vi "GyroSampleSensorLoop.vi"   [LabVIEW 2016]
uses:
  GyroRxLoopData.ctl
  GyroRxLoopStates.ctl
  GyroSBITSample.ctl
  GyroLBITSample.ctl
  GyroSample.ctl
  GyroErrorSample.ctl
  GyroErrorCodes.ctl
  <vilib>/Platform/TimedLoop/XDataNode/timing_clust.ctl
  <vilib>/Platform/TimedLoop/XDataNode/nitl_modes.ctl
  <vilib>/Platform/TimedLoop/XDataNode/wakeup.ctl
  <vilib>/rvi/Emulation/niFpgaSctlEmulationGetInTimedLoop.vi
  <vilib>/rvi/Emulation/niFpgaEmulationReportErrorSimple.vi
  <vilib>/rvi/Emulation/niFpgaGetClockAttributes.vi
  <vilib>/rvi/Emulation/niFpgaCriticalErrorInLSC.vi
  <vilib>/rvi/Emulation/niFpgaEmulationIsFPGAContextNoSignature.vi
  <vilib>/rvi/errors/niFpgaSetErrorForExecOnDevCompSimple.vi
  <vilib>/rvi/eio/common/nirviEmuReportErrorAndStop.vi
  <vilib>/rvi/DataTransferAndStorage/Container/Common/niFpgaContainerGetUniqueNameForEmu.vi
  <vilib>/rvi/FIFO/Fifo_Resource/nirvififoEmulationSetSize.vi
  <vilib>/rvi/FIFO/Fifo_Resource/nirviFifoEmulationQueueMgr.vi
  <instcachedir>/0/nirviFifoEmulationQueueMgr_E5CAEC123FF24DC58D834DCA3CDAA9B5.lvgen/nirviFifoEmulationQueueMgr_E5CAEC123FF24DC58D834DCA3CDAA9B5_009.vi
  <vilib>/Utility/error.llb/Clear Errors.vi
  <vilib>/rvi/FIFO/Fifo_Resource/nirvififoEmulationCreateLock.vi
  <vilib>/rvi/Emulation/niFpgaProcessEmulError.vi
  <vilib>/rvi/FIFO/Fifo_Resource/nirvififoEmulationObtainLock.vi
  <vilib>/rvi/FIFO/Fifo_Resource/nirvififoEmulationReleaseLock.vi
  <vilib>/rvi/occurrence/nirviWaitOnOccurrenceBase.vi
  <vilib>/rvi/errors/nirviReportUnexpectedCaseInternalError.vi
  <vilib>/rvi/errors/nirviReportUnexpectedCaseInternalError (U32).vi
  <vilib>/rvi/FIFO/Fifo_Resource/nirvififoEmulationDetermineInputValidOut.vi
  <vilib>/rvi/Memory/Memory_Emulation/niFpgaMemoryEmulationCacheClearOnFirstRun.vi
  <vilib>/rvi/Memory/Memory_Emulation/nirvimemoryEmulationManagerCache_MakeExclusive.vi
  <vilib>/rvi/Memory/Memory_Emulation/niFpgaMemoryEmulationValidateCache.vi
  <vilib>/rvi/Memory/Memory_Emulation/nirvimemoryEmulationManagerCache_InsertValue.vi
  <vilib>/rvi/Memory/Memory_Emulation/nirvimemoryEmulationManagerCache_ReleaseExclusive.vi
  <vilib>/rvi/Memory/Memory_Emulation/nirvimemoryEmulationManagerCache_GetValue.vi
  <vilib>/rvi/Memory/Memory_Emulation/nirvimemoryEmulationManagerCache_SetValue.vi
  <instcachedir>/0/nirviFifoEmulationQueueMgr_E5CAEC123FF24DC58D834DCA3CDAA9B5.lvgen/nirviFifoEmulationQueueMgr_E5CAEC123FF24DC58D834DCA3CDAA9B5_040.vi
  <instcachedir>/0/nirviFifoEmulationQueueMgr_E5CAEC123FF24DC58D834DCA3CDAA9B5.lvgen/nirviFifoEmulationQueueMgr_E5CAEC123FF24DC58D834DCA3CDAA9B5_041.vi
  <instcachedir>/0/nirviFifoEmulationQueueMgr_E5CAEC123FF24DC58D834DCA3CDAA9B5.lvgen/nirviFifoEmulationQueueMgr_E5CAEC123FF24DC58D834DCA3CDAA9B5_004.vi
  <instcachedir>/0/nirviFifoEmulationQueueMgr_E5CAEC123FF24DC58D834DCA3CDAA9B5.lvgen/nirviFifoEmulationQueueMgr_E5CAEC123FF24DC58D834DCA3CDAA9B5_006.vi
  <instcachedir>/0/nirviFifoEmulationQueueMgr_E5CAEC123FF24DC58D834DCA3CDAA9B5.lvgen/nirviFifoEmulationQueueMgr_E5CAEC123FF24DC58D834DCA3CDAA9B5_042.vi
  <instcachedir>/0/nirviFifoEmulationQueueMgr_E5CAEC123FF24DC58D834DCA3CDAA9B5.lvgen/nirviFifoEmulationQueueMgr_E5CAEC123FF24DC58D834DCA3CDAA9B5_043.vi
  <vilib>/Platform/TimedLoop/XDataNode/XDataNode.xnode
  <vilib>/rvi/DataTransferAndStorage/Container/XNode/niFpgaContainer.xnode
  <vilib>/rvi/FIFO/Fifo_Resource/nirvififoEmulationRead.vi
  <vilib>/rvi/FIFO/Fifo_Resource/nirvififoEmulationWrite.vi
  <vilib>/rvi/DataTransferAndStorage/Register/Emulation/niFpgaRegisterEmulation.vi
  <vilib>/Platform/TimedLoop/XDataNode/XDNodeRunTimeDep.lvlib
types:
  T1 = typedef "GyroRxLoopData.ctl" = cluster{"State":T2, "Timestamp":u64, "Timeout":i32, "CRC":u32, "Checksum":u8, "IsLBIT":bool, "ReservedCount":u8, "SBITSample":T3, "LBITSample":T4, "Sample":T5, "ErrorSample":T6}
  T2 = typedef "GyroRxLoopStates.ctl" = enum16{"ReadHeader3", "IgnoreASCIIResponse", "ReadNormalHeader2", "ReadNormalHeader1", "ReadBITHeader0", "ReadBIT0", "ReadBIT1", "ReadBIT2", "ReadBIT3", "ReadBIT4", "ReadBIT5", "ReadBIT6", "ReadBIT7", "ReadChecksum", "PrepareSBIT", "MoveSBIT", "PrepareLBIT", "MoveLBIT", "ReadSampleHeader0", "ReadSampleX3", "ReadSampleX2", "ReadSampleX1", "ReadSampleX0", "ReadSampleY3", "ReadSampleY2", "ReadSampleY1", "ReadSampleY0", "ReadSampleZ3", "ReadSampleZ2", "ReadSampleZ1", "ReadSampleZ0", "ReadSampleReserved", "ReadSampleStatus", "ReadSampleSequenceNumber", "ReadSampleTemperature1", "ReadSampleTemperature0", "ReadSampleCRC3", "ReadSampleCRC2", "ReadSampleCRC1", "ReadSampleCRC0", "VerifyCRC", "PrepareSample", "MoveSample", "ResponseHeaderError", "ResponseCRCError", "ResponseTimeoutError", "ResponseChecksumError", "PrepareErrorCode", "MoveErrorCode", "ClearCRC", "WaitForCRCCleared"}
  T3 = typedef "GyroSBITSample.ctl" = cluster{"Timestamp":u64, "TxBytes":u64, "RxBytes":u64, "TxFrames":u64, "RxFrames":u64, "BIT0":u8, "BIT1":u8, "BIT2":u8, "BIT3":u8, "BIT4":u8, "BIT5":u8}
  T4 = typedef "GyroLBITSample.ctl" = cluster{"Timestamp":u64, "TxBytes":u64, "RxBytes":u64, "TxFrames":u64, "RxFrames":u64, "BIT0":u8, "BIT1":u8, "BIT2":u8, "BIT3":u8, "BIT4":u8, "BIT5":u8, "BIT6":u8, "BIT7":u8}
  T5 = typedef "GyroSample.ctl" = cluster{"Timestamp":u64, "TxBytes":u64, "RxBytes":u64, "TxFrames":u64, "RxFrames":u64, "GyroX":u32, "GyroY":u32, "GyroZ":u32, "Status":u8, "SequenceNumber":u8, "Temperature":i16}
  T6 = typedef "GyroErrorSample.ctl" = cluster{"Timestamp":u64, "TxBytes":u64, "RxBytes":u64, "TxFrames":u64, "RxFrames":u64, "ErrorCode":T7}
  T7 = typedef "GyroErrorCodes.ctl" = enum8{"None", "ResponseHeaderError", "ResponseCRCError", "ResponseTimeoutError", "ResponseChecksumError"}
  T8 = typedef "XDNodeRunTimeDep.lvlib/timing_clust.ctl" = cluster{"Expected End [f-1]":u64, "Actual End [f-1]":u64, "Finished Late? [f-1]":bool, "Expected End [i-1]":u64, "Actual End [i-1]":u64, "Finished Late? [i-1]":bool, "Expected Start [i]":u64, "Actual Start [i]":u64, "Expected Start [f]":u64, "Actual Start [f]":u64, "Source Name":string, "Structure Name":string, "Period":i64, "Deadline":i64, "Offset":i64, "Start":i64, "Priority":i32, "Timeout":i32, "Mode":T9, "Wakeup Reason":T10, "Error":errorcluster, "Source Type":string, "Secondary Source Type":string, "Global End Time":u64, "Global Start Time":u64, "Frame Duration":u64, "Iteration Duration":u64, "Assigned CPU":i32, "I/O Scan Engine Mode":u32}
  T9 = typedef "XDNodeRunTimeDep.lvlib/nitl_modes.ctl" = enum32{"No Change", "Process missed periods, maintain original phase", "Discard missed periods, maintain original phase", "Process missed periods, ignore original phase", "Discard missed periods, ignore original phase"}
  T10 = typedef "XDNodeRunTimeDep.lvlib/wakeup.ctl" = enum32{"Normal", "Aborted", "Asynchronous wakeup", "Timing source error", "Timed loop error", "Timeout"}
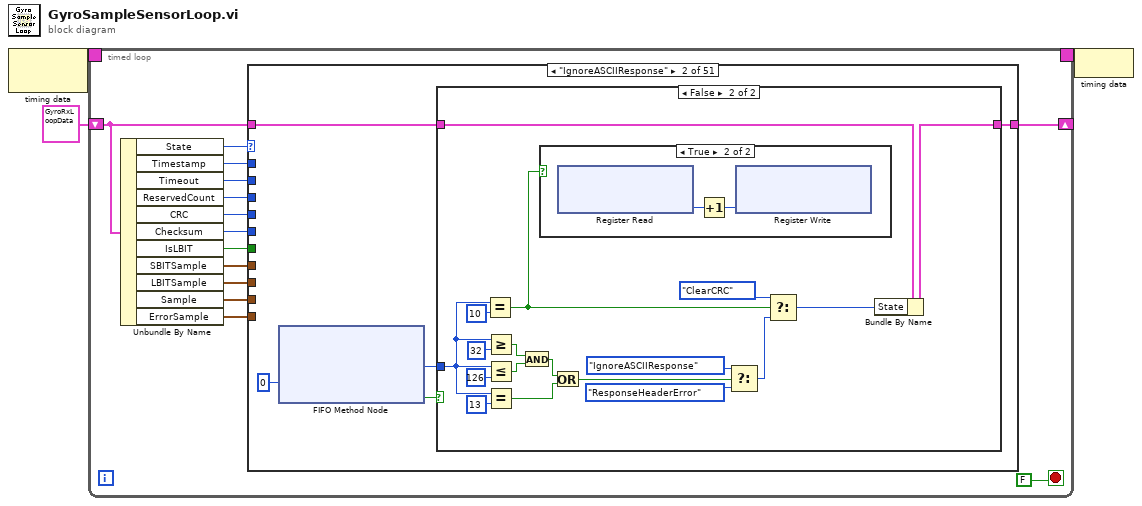
[diagram p0: block diagram]
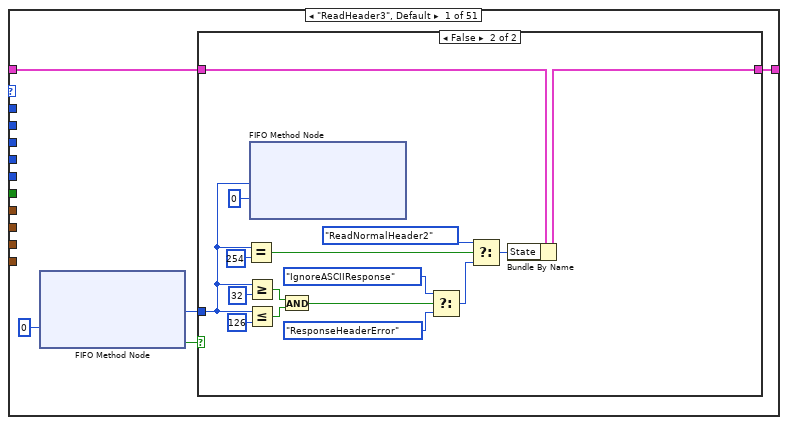
[diagram p2: hidden frame]
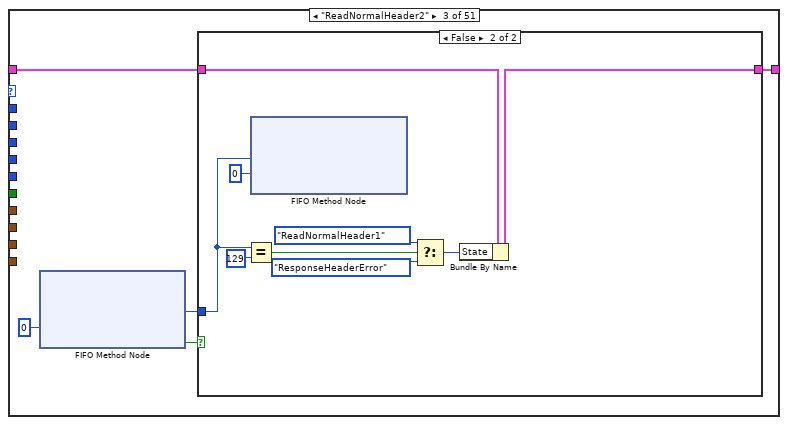
[diagram p6: hidden frame]
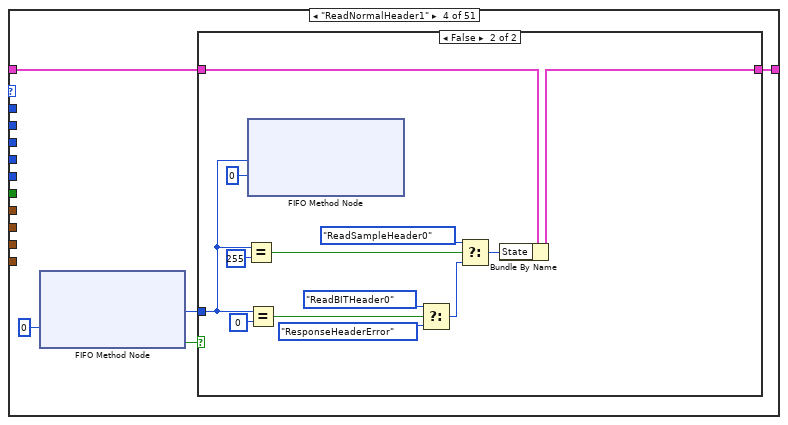
[diagram p8: hidden frame]
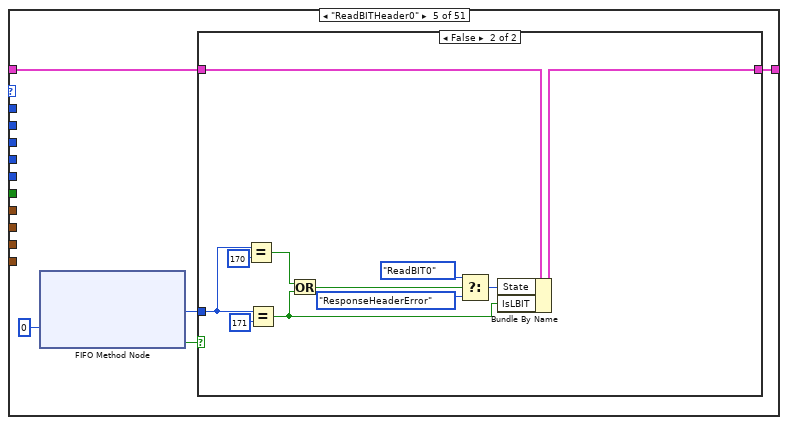
[diagram p10: hidden frame]
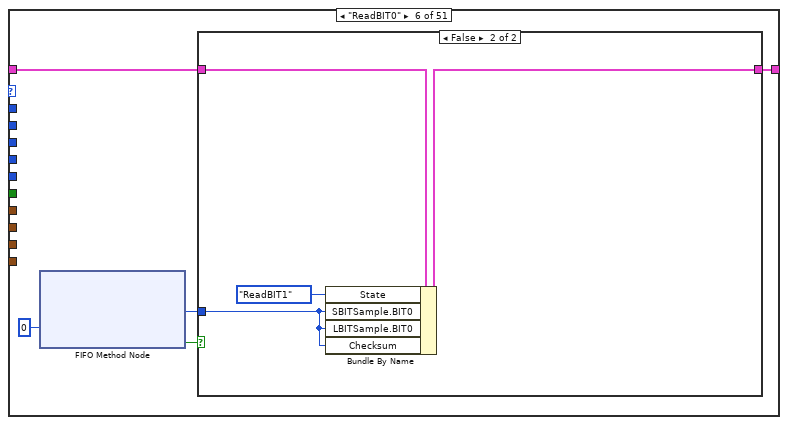
[diagram p12: hidden frame]
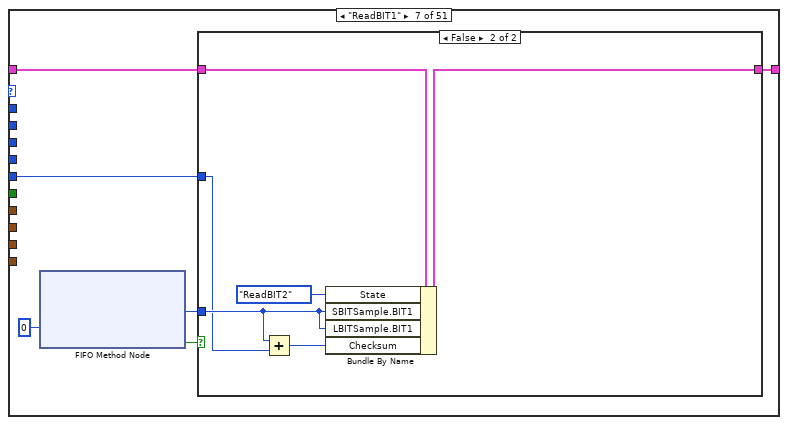
[diagram p14: hidden frame]
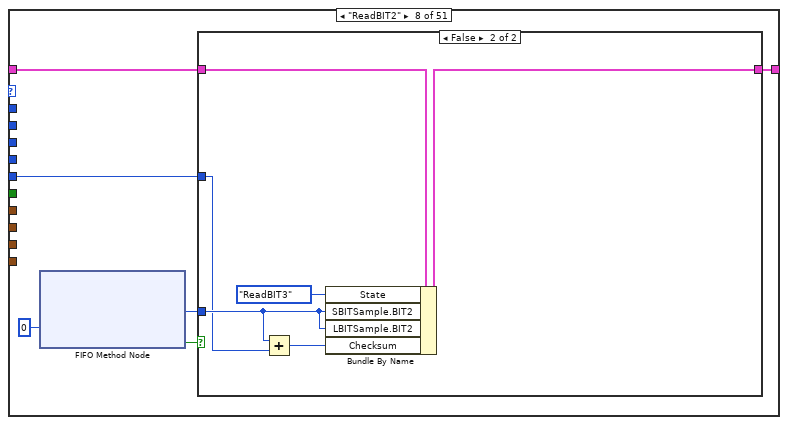
[diagram p16: hidden frame]
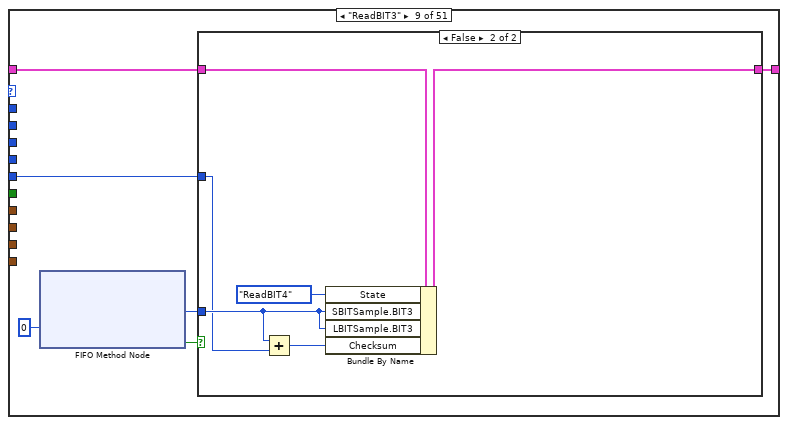
[diagram p18: hidden frame]
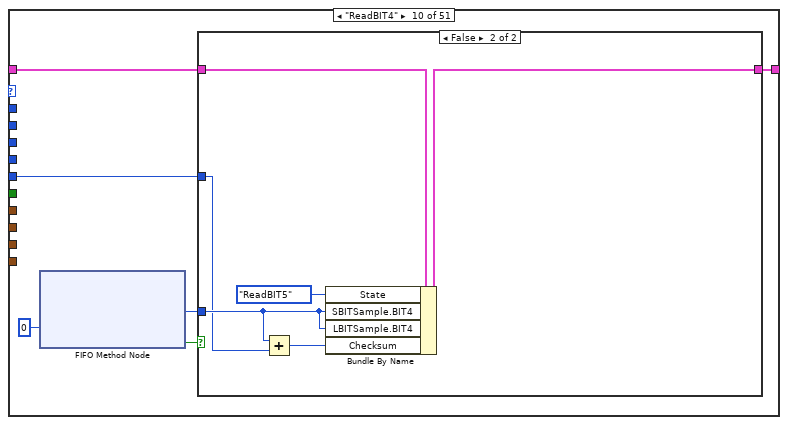
[diagram p20: hidden frame]
diagram:
  n1 = node-c288() -> (w3:T8)  [unwired: 1 in]
  n2 = timed-loop {
    timing: w3 -> [_]
    timing-out: [_] -> w2
    shift-right: [w17] -> _
    shift-left: T1 {"State"=enum."ReadHeader3", "Timestamp"=0, "Timeout"=0, "CRC"=0, "Checksum"=0, "IsLBIT"=FALSE, "ReservedCount"=0, "SBITSample"={"Timestamp"=0, "TxBytes"=0, "RxBytes"=0, "TxFrames"=0, "RxFrames"=0, "BIT0"=0, "BIT1"=0, "BIT2"=0, "BIT3"=0, "BIT4"=0, "BIT5"=0}, "LBITSample"={"Timestamp"=0, "TxBytes"=0, "RxBytes"=0, "TxFrames"=0, "RxFrames"=0, "BIT0"=0, "BIT1"=0, "BIT2"=0, "BIT3"=0, "BIT4"=0, "BIT5"=0, "BIT6"=0, "BIT7"=0}, "Sample"={"Timestamp"=0, "TxBytes"=0, "RxBytes"=0, "TxFrames"=0, "RxFrames"=0, "GyroX"=0, "GyroY"=0, "GyroZ"=0, "Status"=0, "SequenceNumber"=0, "Temperature"=0}, "ErrorSample"={"Timestamp"=0, "TxBytes"=0, "RxBytes"=0, "TxFrames"=0, "RxFrames"=0, "ErrorCode"=enum."None"}} ("GyroRxLoopData") -> [w16]
    stop <- FALSE stop-if-true
    n3 = Unbundle By Name(w16) -> ("State"=w15:T2, "Timestamp"=w14:u64, "Timeout"=w13:i32, "ReservedCount"=w9:u8, "CRC"=w12:u32, "Checksum"=w11:u8, "IsLBIT"=w10:bool, "SBITSample"=w8:T3, "LBITSample"=w7:T4, "Sample"=w6:T5, "ErrorSample"=w5:T6)
    n4 = case shown="\"IgnoreASCIIResponse\"" w15 {
      tunnel: [w18 w40 w66 w81 w100 w117 w128 w141 w154 w167 w181 w197 w210 w224 w249 w254 w262 w267 w269 w284 w298 w314 w330 w344 w358 w374 w390 w404 w418 w434 w450 w466 w483 w494 w505 w519 w533 w549 w565 w581 w595 w617 w622 w626 w630 w634 w638 w646 w651 w656 w663] -> w17
      tunnel: w16 -> [w19 w41 w67 w82 w101 w118 w129 w142 w155 w168 w182 w198 w211 w225 w250 w255 w263 w268 w270 w285 w299 w315 w331 w345 w359 w375 w391 w405 w419 w435 w451 w467 w484 w495 w506 w520 w534 w550 w566 w582 w596 w618 w623 w627 w631 w635 w639 w647 w652 w657 w664]
      tunnel: w14 -> [_ _ _ _ _ _ _ _ _ _ _ _ _ _ w247 _ w260 _ _ _ _ _ _ _ _ _ _ _ _ _ _ _ _ _ _ _ _ _ _ _ _ w615 _ _ _ _ _ w644 _ _ _]
      tunnel: w13 -> [_ _ _ _ _ _ _ _ _ _ _ _ _ _ _ _ _ _ _ _ _ _ _ _ _ _ _ _ _ _ _ _ _ _ _ _ _ _ _ _ _ _ _ _ _ _ _ _ _ _ _]
      tunnel: w12 -> [_ _ _ _ _ _ _ _ _ _ _ _ _ _ _ _ _ _ _ _ _ _ _ _ _ _ _ _ _ _ _ _ _ _ _ _ _ w548 w564 w580 w594 _ _ _ _ _ _ _ _ _ _]
      tunnel: w11 -> [_ _ _ _ _ _ w127 w140 w153 w166 w180 w196 w209 w223 _ _ _ _ _ _ _ _ _ _ _ _ _ _ _ _ _ _ _ _ _ _ _ _ _ _ _ _ _ _ _ _ _ _ _ _ _]
      tunnel: w10 -> [_ _ _ _ _ _ _ _ _ _ w179 _ _ w222 _ _ _ _ _ _ _ _ _ _ _ _ _ _ _ _ _ _ _ _ _ _ _ _ _ _ _ _ _ _ _ _ _ _ _ _ _]
      tunnel: w9 -> [_ _ _ _ _ _ _ _ _ _ _ _ _ _ _ _ _ _ _ _ _ _ _ _ _ _ _ _ _ _ _ w465 _ _ _ _ _ _ _ _ _ _ _ _ _ _ _ _ _ _ _]
      tunnel: w8 -> [_ _ _ _ _ _ _ _ _ _ _ _ _ _ _ w251 _ _ _ _ _ _ _ _ _ _ _ _ _ _ _ _ _ _ _ _ _ _ _ _ _ _ _ _ _ _ _ _ _ _ _]
      tunnel: w7 -> [_ _ _ _ _ _ _ _ _ _ _ _ _ _ _ _ _ w264 _ _ _ _ _ _ _ _ _ _ _ _ _ _ _ _ _ _ _ _ _ _ _ _ _ _ _ _ _ _ _ _ _]
      tunnel: w6 -> [_ _ _ _ _ _ _ _ _ _ _ _ _ _ _ _ _ _ _ _ _ _ _ _ _ _ _ _ _ _ _ _ _ _ _ _ _ _ _ _ _ _ w620 _ _ _ _ _ _ _ _]
      tunnel: w5 -> [_ _ _ _ _ _ _ _ _ _ _ _ _ _ _ _ _ _ _ _ _ _ _ _ _ _ _ _ _ _ _ _ _ _ _ _ _ _ _ _ _ _ _ _ _ _ _ _ w649 _ _]
      frame "ReadHeader3", Default {
        n5 = xnode ("FIFO Method Node")("Timeout"=0) -> ("Element"=w21:u8, "Timed Out?"=w20:bool)  [unwired: 1 in, 1 out]
        n6 = case shown="False" w20 {
          tunnel: w21 -> [_ w25]
          tunnel: w19 -> [w23 w28]
          tunnel: [w23 w27] -> w18
          frame True {
          }
          frame False {
            n7 = Equal?(x=w25, y=u8 254) -> (x = y?=w29:bool)
            n8 = Greater Or Equal?(x=w25, y=u8 32) -> (x >= y?=w36:bool)
            n9 = Less Or Equal?(x=w25, y=u8 126) -> (x <= y?=w35:bool)
            n10 = xnode ("FIFO Method Node")("Element"=w25, "Timeout"=0) -> ()  [unwired: 1 in, 2 out]
            n11 = And(x=w36, y=w35) -> (x .and. y?=w34:bool)
            n12 = Select(t=GyroRxLoopStates."IgnoreASCIIResponse", s=w34, f=GyroRxLoopStates."ResponseHeaderError" ("GyroRxLoopStates")) -> (s? t:f=w33:T2)
            n13 = Select(t=GyroRxLoopStates."ReadNormalHeader2", s=w29, f=w33) -> (s? t:f=w26:T2)
            n14 = Bundle By Name(cluster=w28, "State"=w26) -> (w27:T1)
          }
        }
      }
      frame "IgnoreASCIIResponse" {
        n15 = xnode ("FIFO Method Node")("Timeout"=0) -> ("Element"=w43:u8, "Timed Out?"=w42:bool)  [unwired: 1 in, 1 out]
        n16 = case shown="False" w42 {
          tunnel: w43 -> [_ w55]
          tunnel: w41 -> [w45 w59]
          tunnel: [w45 w58] -> w40
          frame True {
          }
          frame False {
            n17 = Equal?(x=w55, y=u8 10) -> (x = y?=w46:bool)
            n18 = Greater Or Equal?(x=w55, y=u8 32) -> (x >= y?=w54:bool)
            n19 = Less Or Equal?(x=w55, y=u8 126) -> (x <= y?=w53:bool)
            n20 = Equal?(x=w55, y=u8 13) -> (x = y?=w51:bool)
            n21 = And(x=w54, y=w53) -> (x .and. y?=w52:bool)
            n22 = case shown="True" w46 {
              frame False {
              }
              frame True {
                n23 = xnode ("Register Read")() -> ("Data"=w65:u64)  [unwired: 1 in, 1 out]
                n24 = Increment(x=w65) -> (x+1=w64:u64)
                n25 = xnode ("Register Write")("Data"=w64) -> ()  [unwired: 1 in, 1 out]
              }
            }
            n26 = Or(x=w52, y=w51) -> (x .or. y?=w50:bool)
            n27 = Select(t=GyroRxLoopStates."IgnoreASCIIResponse", s=w50, f=GyroRxLoopStates."ResponseHeaderError" ("t")) -> (s? t:f=w47:T2)
            n28 = Select(t=GyroRxLoopStates."ClearCRC", s=w46, f=w47) -> (s? t:f=w57:T2)
            n29 = Bundle By Name(cluster=w59, "State"=w57) -> (w58:T1)
          }
        }
      }
      frame "ReadNormalHeader2" {
        n30 = xnode ("FIFO Method Node")("Timeout"=0) -> ("Element"=w69:u8, "Timed Out?"=w68:bool)  [unwired: 1 in, 1 out]
        n31 = case shown="False" w68 {
          tunnel: w69 -> [_ w72]
          tunnel: w67 -> [w71 w77]
          tunnel: [w71 w76] -> w66
          frame True {
          }
          frame False {
            n32 = Equal?(x=w72, y=u8 129) -> (x = y?=w78:bool)
            n33 = xnode ("FIFO Method Node")("Element"=w72, "Timeout"=0) -> ()  [unwired: 1 in, 2 out]
            n34 = Select(t=GyroRxLoopStates."ReadNormalHeader1", s=w78, f=GyroRxLoopStates."ResponseHeaderError") -> (s? t:f=w75:T2)
            n35 = Bundle By Name(cluster=w77, "State"=w75) -> (w76:T1)
          }
        }
      }
      frame "ReadNormalHeader1" {
        n36 = xnode ("FIFO Method Node")("Timeout"=0) -> ("Element"=w84:u8, "Timed Out?"=w83:bool)  [unwired: 1 in, 1 out]
        n37 = case shown="False" w83 {
          tunnel: w84 -> [_ w87]
          tunnel: w82 -> [w86 w96]
          tunnel: [w86 w95] -> w81
          frame True {
          }
          frame False {
            n38 = Equal?(x=w87, y=u8 255) -> (x = y?=w97:bool)
            n39 = xnode ("FIFO Method Node")("Element"=w87, "Timeout"=0) -> ()  [unwired: 1 in, 2 out]
            n40 = Equal?(x=w87, y=u8 0) -> (x = y?=w92:bool)
            n41 = Select(t=GyroRxLoopStates."ReadBITHeader0" ("f"), s=w92, f=GyroRxLoopStates."ResponseHeaderError") -> (s? t:f=w89:T2)
            n42 = Select(t=GyroRxLoopStates."ReadSampleHeader0", s=w97, f=w89) -> (s? t:f=w94:T2)
            n43 = Bundle By Name(cluster=w96, "State"=w94) -> (w95:T1)
          }
        }
      }
      frame "ReadBITHeader0" {
        n44 = xnode ("FIFO Method Node")("Timeout"=0) -> ("Element"=w103:u8, "Timed Out?"=w102:bool)  [unwired: 1 in, 1 out]
        n45 = case shown="False" w102 {
          tunnel: w103 -> [_ w110]
          tunnel: w101 -> [w105 w114]
          tunnel: [w105 w113] -> w100
          frame True {
          }
          frame False {
            n46 = Equal?(x=w110, y=u8 170) -> (x = y?=w109:bool)
            n47 = Equal?(x=w110, y=u8 171) -> (x = y?=w107:bool)
            n48 = Or(x=w109, y=w107) -> (x .or. y?=w108:bool)
            n49 = Select(t=GyroRxLoopStates."ReadBIT0", s=w108, f=GyroRxLoopStates."ResponseHeaderError") -> (s? t:f=w112:T2)
            n50 = Bundle By Name(cluster=w114, "State"=w112, "IsLBIT"=w107) -> (w113:T1)
          }
        }
      }
      frame "ReadBIT0" {
        n51 = xnode ("FIFO Method Node")("Timeout"=0) -> ("Element"=w120:u8, "Timed Out?"=w119:bool)  [unwired: 1 in, 1 out]
        n52 = case shown="False" w119 {
          tunnel: w120 -> [_ w123]
          tunnel: w118 -> [w122 w126]
          tunnel: [w122 w125] -> w117
          frame True {
          }
          frame False {
            n53 = Bundle By Name(cluster=w126, "State"=GyroRxLoopStates."ReadBIT1" ("t"), "SBITSample.BIT0"=w123, "LBITSample.BIT0"=w123, "Checksum"=w123) -> (w125:T1)
          }
        }
      }
      frame "ReadBIT1" {
        n54 = xnode ("FIFO Method Node")("Timeout"=0) -> ("Element"=w131:u8, "Timed Out?"=w130:bool)  [unwired: 1 in, 1 out]
        n55 = case shown="False" w130 {
          tunnel: w131 -> [_ w136]
          tunnel: w129 -> [w133 w139]
          tunnel: [w133 w138] -> w128
          tunnel: w127 -> [_ w135]
          frame True {
          }
          frame False {
            n56 = Add(x=w136, y=w135) -> (x+y=w134:u8)
            n57 = Bundle By Name(cluster=w139, "State"=GyroRxLoopStates."ReadBIT2" ("t"), "SBITSample.BIT1"=w136, "LBITSample.BIT1"=w136, "Checksum"=w134) -> (w138:T1)
          }
        }
      }
      frame "ReadBIT2" {
        n58 = xnode ("FIFO Method Node")("Timeout"=0) -> ("Element"=w144:u8, "Timed Out?"=w143:bool)  [unwired: 1 in, 1 out]
        n59 = case shown="False" w143 {
          tunnel: w144 -> [_ w149]
          tunnel: w142 -> [w146 w152]
          tunnel: [w146 w151] -> w141
          tunnel: w140 -> [_ w148]
          frame True {
          }
          frame False {
            n60 = Add(x=w149, y=w148) -> (x+y=w147:u8)
            n61 = Bundle By Name(cluster=w152, "State"=GyroRxLoopStates."ReadBIT3" ("t"), "SBITSample.BIT2"=w149, "LBITSample.BIT2"=w149, "Checksum"=w147) -> (w151:T1)
          }
        }
      }
      frame "ReadBIT3" {
        n62 = xnode ("FIFO Method Node")("Timeout"=0) -> ("Element"=w157:u8, "Timed Out?"=w156:bool)  [unwired: 1 in, 1 out]
        n63 = case shown="False" w156 {
          tunnel: w157 -> [_ w162]
          tunnel: w155 -> [w159 w165]
          tunnel: [w159 w164] -> w154
          tunnel: w153 -> [_ w161]
          frame True {
          }
          frame False {
            n64 = Add(x=w162, y=w161) -> (x+y=w160:u8)
            n65 = Bundle By Name(cluster=w165, "State"=GyroRxLoopStates."ReadBIT4" ("t"), "SBITSample.BIT3"=w162, "LBITSample.BIT3"=w162, "Checksum"=w160) -> (w164:T1)
          }
        }
      }
      frame "ReadBIT4" {
        n66 = xnode ("FIFO Method Node")("Timeout"=0) -> ("Element"=w170:u8, "Timed Out?"=w169:bool)  [unwired: 1 in, 1 out]
        n67 = case shown="False" w169 {
          tunnel: w170 -> [_ w175]
          tunnel: w168 -> [w172 w178]
          tunnel: [w172 w177] -> w167
          tunnel: w166 -> [_ w174]
          frame True {
          }
          frame False {
            n68 = Add(x=w175, y=w174) -> (x+y=w173:u8)
            n69 = Bundle By Name(cluster=w178, "State"=GyroRxLoopStates."ReadBIT5" ("t"), "SBITSample.BIT4"=w175, "LBITSample.BIT4"=w175, "Checksum"=w173) -> (w177:T1)
          }
        }
      }
      frame "ReadBIT5" {
        n70 = xnode ("FIFO Method Node")("Timeout"=0) -> ("Element"=w184:u8, "Timed Out?"=w183:bool)  [unwired: 1 in, 1 out]
        n71 = case shown="False" w183 {
          tunnel: w184 -> [_ w193]
          tunnel: w182 -> [w186 w195]
          tunnel: [w186 w194] -> w181
          tunnel: w180 -> [_ w192]
          tunnel: w179 -> [_ w190]
          frame True {
          }
          frame False {
            n72 = Add(x=w193, y=w192) -> (x+y=w191:u8)
            n73 = Select(t=GyroRxLoopStates."ReadBIT6", s=w190, f=GyroRxLoopStates."ReadChecksum") -> (s? t:f=w187:T2)
            n74 = Bundle By Name(cluster=w195, "State"=w187, "SBITSample.BIT5"=w193, "LBITSample.BIT5"=w193, "Checksum"=w191) -> (w194:T1)
          }
        }
      }
      frame "ReadBIT6" {
        n75 = xnode ("FIFO Method Node")("Timeout"=0) -> ("Element"=w200:u8, "Timed Out?"=w199:bool)  [unwired: 1 in, 1 out]
        n76 = case shown="False" w199 {
          tunnel: w200 -> [_ w206]
          tunnel: w198 -> [w202 w208]
          tunnel: [w202 w207] -> w197
          tunnel: w196 -> [_ w205]
          frame True {
          }
          frame False {
            n77 = Add(x=w206, y=w205) -> (x+y=w204:u8)
            n78 = Bundle By Name(cluster=w208, "State"=GyroRxLoopStates."ReadBIT7" ("t"), "LBITSample.BIT6"=w206, "Checksum"=w204) -> (w207:T1)
          }
        }
      }
      frame "ReadBIT7" {
        n79 = xnode ("FIFO Method Node")("Timeout"=0) -> ("Element"=w213:u8, "Timed Out?"=w212:bool)  [unwired: 1 in, 1 out]
        n80 = case shown="False" w212 {
          tunnel: w213 -> [_ w219]
          tunnel: w211 -> [w215 w221]
          tunnel: [w215 w220] -> w210
          tunnel: w209 -> [_ w218]
          frame True {
          }
          frame False {
            n81 = Add(x=w219, y=w218) -> (x+y=w217:u8)
            n82 = Bundle By Name(cluster=w221, "State"=GyroRxLoopStates."ReadChecksum" ("t"), "LBITSample.BIT7"=w219, "Checksum"=w217) -> (w220:T1)
          }
        }
      }
      frame "ReadChecksum" {
        n83 = xnode ("FIFO Method Node")("Timeout"=0) -> ("Element"=w227:u8, "Timed Out?"=w226:bool)  [unwired: 1 in, 1 out]
        n84 = case shown="False" w226 {
          tunnel: w227 -> [_ w238]
          tunnel: w225 -> [w229 w240]
          tunnel: [w229 w239] -> w224
          tunnel: w223 -> [_ w237]
          tunnel: w222 -> [_ w236]
          frame True {
          }
          frame False {
            n85 = Not Equal?(x=w237, y=w238) -> (x != y?=w230:bool)
            n86 = Select(t=GyroRxLoopStates."PrepareLBIT", s=w236, f=GyroRxLoopStates."PrepareSBIT" ("t")) -> (s? t:f=w232:T2)
            n87 = case shown="False" w230 {
              frame True {
              }
              frame False {
                n88 = xnode ("Register Read")() -> ("Data"=w242:u64)  [unwired: 1 in, 1 out]
                n89 = Increment(x=w242) -> (x+1=w241:u64)
                n90 = xnode ("Register Write")("Data"=w241) -> ()  [unwired: 1 in, 1 out]
              }
            }
            n91 = Select(t=GyroRxLoopStates."ResponseChecksumError", s=w230, f=w232) -> (s? t:f=w231:T2)
            n92 = Bundle By Name(cluster=w240, "State"=w231) -> (w239:T1)
          }
        }
      }
      frame "PrepareSBIT" {
        n93 = xnode ("Register Read")() -> ("Data"=w246:u64)  [unwired: 1 in, 1 out]
        n94 = xnode ("Register Read")() -> ("Data"=w245:u64)  [unwired: 1 in, 1 out]
        n95 = xnode ("Register Read")() -> ("Data"=w244:u64)  [unwired: 1 in, 1 out]
        n96 = xnode ("Register Read")() -> ("Data"=w243:u64)  [unwired: 1 in, 1 out]
        n97 = Bundle By Name(cluster=w250, "State"=GyroRxLoopStates."MoveSBIT", "SBITSample.Timestamp"=w247, "SBITSample.TxBytes"=w246, "SBITSample.RxBytes"=w245, "SBITSample.TxFrames"=w244, "SBITSample.RxFrames"=w243) -> (w249:T1)
      }
      frame "MoveSBIT" {
        n98 = xnode ("FIFO Method Node")("Element"=w251, "Timeout"=0) -> ()  [unwired: 1 in, 2 out]
        n99 = Bundle By Name(cluster=w255, "State"=GyroRxLoopStates."ClearCRC") -> (w254:T1)
      }
      frame "PrepareLBIT" {
        n100 = xnode ("Register Read")() -> ("Data"=w259:u64)  [unwired: 1 in, 1 out]
        n101 = xnode ("Register Read")() -> ("Data"=w258:u64)  [unwired: 1 in, 1 out]
        n102 = xnode ("Register Read")() -> ("Data"=w257:u64)  [unwired: 1 in, 1 out]
        n103 = xnode ("Register Read")() -> ("Data"=w256:u64)  [unwired: 1 in, 1 out]
        n104 = Bundle By Name(cluster=w263, "State"=GyroRxLoopStates."MoveLBIT", "LBITSample.Timestamp"=w260, "LBITSample.TxBytes"=w259, "LBITSample.RxBytes"=w258, "LBITSample.TxFrames"=w257, "LBITSample.RxFrames"=w256) -> (w262:T1)
      }
      frame "MoveLBIT" {
        n105 = xnode ("FIFO Method Node")("Element"=w264, "Timeout"=0) -> ()  [unwired: 1 in, 2 out]
        n106 = Bundle By Name(cluster=w268, "State"=GyroRxLoopStates."ClearCRC") -> (w267:T1)
      }
      frame "ReadSampleHeader0" {
        n107 = xnode ("FIFO Method Node")("Timeout"=0) -> ("Element"=w272:u8, "Timed Out?"=w271:bool)  [unwired: 1 in, 1 out]
        n108 = case shown="False" w271 {
          tunnel: w272 -> [_ w275]
          tunnel: w270 -> [w274 w281]
          tunnel: [w274 w280] -> w269
          frame True {
          }
          frame False {
            n109 = xnode ("FIFO Method Node")("Element"=w275, "Timeout"=0) -> ()  [unwired: 1 in, 2 out]
            n110 = Equal?(x=w275, y=u8 85) -> (x = y?=w277:bool)
            n111 = Select(t=GyroRxLoopStates."ReadSampleX3", s=w277, f=GyroRxLoopStates."ResponseHeaderError") -> (s? t:f=w279:T2)
            n112 = Bundle By Name(cluster=w281, "State"=w279) -> (w280:T1)
          }
        }
      }
      frame "ReadSampleX3" {
        n113 = xnode ("FIFO Method Node")("Timeout"=0) -> ("Element"=w287:u8, "Timed Out?"=w286:bool)  [unwired: 1 in, 1 out]
        n114 = case shown="False" w286 {
          tunnel: w287 -> [_ w294]
          tunnel: w285 -> [w289 w291]
          tunnel: [w289 w297] -> w284
          frame True {
          }
          frame False {
            n115 = To Unsigned Long Integer(number=w294) -> (unsigned 32bit integer=w293:u32)
            n116 = xnode ("FIFO Method Node")("Element"=w294, "Timeout"=0) -> ()  [unwired: 1 in, 2 out]
            n117 = Logical Shift(y=i16 24, x=w293) -> (x << y=w290:u32)
            n118 = Bundle By Name(cluster=w291, "State"=GyroRxLoopStates."ReadSampleX2" ("t"), "Sample.GyroX"=w290) -> (w297:T1)
          }
        }
      }
      frame "ReadSampleX2" {
        n119 = xnode ("FIFO Method Node")("Timeout"=0) -> ("Element"=w301:u8, "Timed Out?"=w300:bool)  [unwired: 1 in, 1 out]
        n120 = case shown="False" w300 {
          tunnel: w301 -> [_ w310]
          tunnel: w299 -> [w303 w307]
          tunnel: [w303 w313] -> w298
          frame True {
          }
          frame False {
            n121 = Unbundle By Name(w307) -> ("Sample.GyroX"=w306:u32)
            n122 = To Unsigned Long Integer(number=w310) -> (unsigned 32bit integer=w309:u32)
            n123 = xnode ("FIFO Method Node")("Element"=w310, "Timeout"=0) -> ()  [unwired: 1 in, 2 out]
            n124 = Logical Shift(y=i16 16, x=w309) -> (x << y=w305:u32)
            n125 = Or(x=w306, y=w305) -> (x .or. y?=w304:u32)
            n126 = Bundle By Name(cluster=w307, "State"=GyroRxLoopStates."ReadSampleX1" ("t"), "Sample.GyroX"=w304) -> (w313:T1)
          }
        }
      }
      frame "ReadSampleX1" {
        n127 = xnode ("FIFO Method Node")("Timeout"=0) -> ("Element"=w317:u8, "Timed Out?"=w316:bool)  [unwired: 1 in, 1 out]
        n128 = case shown="False" w316 {
          tunnel: w317 -> [_ w326]
          tunnel: w315 -> [w319 w323]
          tunnel: [w319 w329] -> w314
          frame True {
          }
          frame False {
            n129 = Unbundle By Name(w323) -> ("Sample.GyroX"=w322:u32)
            n130 = To Unsigned Long Integer(number=w326) -> (unsigned 32bit integer=w325:u32)
            n131 = xnode ("FIFO Method Node")("Element"=w326, "Timeout"=0) -> ()  [unwired: 1 in, 2 out]
            n132 = Logical Shift(y=i16 8, x=w325) -> (x << y=w321:u32)
            n133 = Or(x=w322, y=w321) -> (x .or. y?=w320:u32)
            n134 = Bundle By Name(cluster=w323, "State"=GyroRxLoopStates."ReadSampleX0" ("t"), "Sample.GyroX"=w320) -> (w329:T1)
          }
        }
      }
      frame "ReadSampleX0" {
        n135 = xnode ("FIFO Method Node")("Timeout"=0) -> ("Element"=w333:u8, "Timed Out?"=w332:bool)  [unwired: 1 in, 1 out]
        n136 = case shown="False" w332 {
          tunnel: w333 -> [_ w340]
          tunnel: w331 -> [w335 w339]
          tunnel: [w335 w343] -> w330
          frame True {
          }
          frame False {
            n137 = Unbundle By Name(w339) -> ("Sample.GyroX"=w338:u32)
            n138 = To Unsigned Long Integer(number=w340) -> (unsigned 32bit integer=w337:u32)
            n139 = xnode ("FIFO Method Node")("Element"=w340, "Timeout"=0) -> ()  [unwired: 1 in, 2 out]
            n140 = Or(x=w338, y=w337) -> (x .or. y?=w336:u32)
            n141 = Bundle By Name(cluster=w339, "State"=GyroRxLoopStates."ReadSampleY3" ("t"), "Sample.GyroX"=w336) -> (w343:T1)
          }
        }
      }
      frame "ReadSampleY3" {
        n142 = xnode ("FIFO Method Node")("Timeout"=0) -> ("Element"=w347:u8, "Timed Out?"=w346:bool)  [unwired: 1 in, 1 out]
        n143 = case shown="False" w346 {
          tunnel: w347 -> [_ w354]
          tunnel: w345 -> [w349 w351]
          tunnel: [w349 w357] -> w344
          frame True {
          }
          frame False {
            n144 = To Unsigned Long Integer(number=w354) -> (unsigned 32bit integer=w353:u32)
            n145 = xnode ("FIFO Method Node")("Element"=w354, "Timeout"=0) -> ()  [unwired: 1 in, 2 out]
            n146 = Logical Shift(y=i16 24, x=w353) -> (x << y=w350:u32)
            n147 = Bundle By Name(cluster=w351, "State"=GyroRxLoopStates."ReadSampleY2" ("t"), "Sample.GyroY"=w350) -> (w357:T1)
          }
        }
      }
      frame "ReadSampleY2" {
        n148 = xnode ("FIFO Method Node")("Timeout"=0) -> ("Element"=w361:u8, "Timed Out?"=w360:bool)  [unwired: 1 in, 1 out]
        n149 = case shown="False" w360 {
          tunnel: w361 -> [_ w370]
          tunnel: w359 -> [w363 w367]
          tunnel: [w363 w373] -> w358
          frame True {
          }
          frame False {
            n150 = Unbundle By Name(w367) -> ("Sample.GyroY"=w366:u32)
            n151 = To Unsigned Long Integer(number=w370) -> (unsigned 32bit integer=w369:u32)
            n152 = xnode ("FIFO Method Node")("Element"=w370, "Timeout"=0) -> ()  [unwired: 1 in, 2 out]
            n153 = Logical Shift(y=i16 16, x=w369) -> (x << y=w365:u32)
            n154 = Or(x=w366, y=w365) -> (x .or. y?=w364:u32)
            n155 = Bundle By Name(cluster=w367, "State"=GyroRxLoopStates."ReadSampleY1" ("t"), "Sample.GyroY"=w364) -> (w373:T1)
          }
        }
      }
      frame "ReadSampleY1" {
        n156 = xnode ("FIFO Method Node")("Timeout"=0) -> ("Element"=w377:u8, "Timed Out?"=w376:bool)  [unwired: 1 in, 1 out]
        n157 = case shown="False" w376 {
          tunnel: w377 -> [_ w386]
          tunnel: w375 -> [w379 w383]
          tunnel: [w379 w389] -> w374
          frame True {
          }
          frame False {
            n158 = Unbundle By Name(w383) -> ("Sample.GyroY"=w382:u32)
            n159 = To Unsigned Long Integer(number=w386) -> (unsigned 32bit integer=w385:u32)
            n160 = xnode ("FIFO Method Node")("Element"=w386, "Timeout"=0) -> ()  [unwired: 1 in, 2 out]
            n161 = Logical Shift(y=i16 8, x=w385) -> (x << y=w381:u32)
            n162 = Or(x=w382, y=w381) -> (x .or. y?=w380:u32)
            n163 = Bundle By Name(cluster=w383, "State"=GyroRxLoopStates."ReadSampleY0" ("t"), "Sample.GyroY"=w380) -> (w389:T1)
          }
        }
      }
      frame "ReadSampleY0" {
        n164 = xnode ("FIFO Method Node")("Timeout"=0) -> ("Element"=w393:u8, "Timed Out?"=w392:bool)  [unwired: 1 in, 1 out]
        n165 = case shown="False" w392 {
          tunnel: w393 -> [_ w400]
          tunnel: w391 -> [w395 w399]
          tunnel: [w395 w403] -> w390
          frame True {
          }
          frame False {
            n166 = Unbundle By Name(w399) -> ("Sample.GyroY"=w398:u32)
            n167 = To Unsigned Long Integer(number=w400) -> (unsigned 32bit integer=w397:u32)
            n168 = xnode ("FIFO Method Node")("Element"=w400, "Timeout"=0) -> ()  [unwired: 1 in, 2 out]
            n169 = Or(x=w398, y=w397) -> (x .or. y?=w396:u32)
            n170 = Bundle By Name(cluster=w399, "State"=GyroRxLoopStates."ReadSampleZ3" ("t"), "Sample.GyroY"=w396) -> (w403:T1)
          }
        }
      }
      frame "ReadSampleZ3" {
        n171 = xnode ("FIFO Method Node")("Timeout"=0) -> ("Element"=w407:u8, "Timed Out?"=w406:bool)  [unwired: 1 in, 1 out]
        n172 = case shown="False" w406 {
          tunnel: w407 -> [_ w414]
          tunnel: w405 -> [w409 w411]
          tunnel: [w409 w417] -> w404
          frame True {
          }
          frame False {
            n173 = To Unsigned Long Integer(number=w414) -> (unsigned 32bit integer=w413:u32)
            n174 = xnode ("FIFO Method Node")("Element"=w414, "Timeout"=0) -> ()  [unwired: 1 in, 2 out]
            n175 = Logical Shift(y=i16 24, x=w413) -> (x << y=w410:u32)
            n176 = Bundle By Name(cluster=w411, "State"=GyroRxLoopStates."ReadSampleZ2" ("t"), "Sample.GyroZ"=w410) -> (w417:T1)
          }
        }
      }
      frame "ReadSampleZ2" {
        n177 = xnode ("FIFO Method Node")("Timeout"=0) -> ("Element"=w421:u8, "Timed Out?"=w420:bool)  [unwired: 1 in, 1 out]
        n178 = case shown="False" w420 {
          tunnel: w421 -> [_ w430]
          tunnel: w419 -> [w423 w427]
          tunnel: [w423 w433] -> w418
          frame True {
          }
          frame False {
            n179 = Unbundle By Name(w427) -> ("Sample.GyroZ"=w426:u32)
            n180 = To Unsigned Long Integer(number=w430) -> (unsigned 32bit integer=w429:u32)
            n181 = xnode ("FIFO Method Node")("Element"=w430, "Timeout"=0) -> ()  [unwired: 1 in, 2 out]
            n182 = Logical Shift(y=i16 16, x=w429) -> (x << y=w425:u32)
            n183 = Or(x=w426, y=w425) -> (x .or. y?=w424:u32)
            n184 = Bundle By Name(cluster=w427, "State"=GyroRxLoopStates."ReadSampleZ1" ("t"), "Sample.GyroZ"=w424) -> (w433:T1)
          }
        }
      }
      frame "ReadSampleZ1" {
        n185 = xnode ("FIFO Method Node")("Timeout"=0) -> ("Element"=w437:u8, "Timed Out?"=w436:bool)  [unwired: 1 in, 1 out]
        n186 = case shown="False" w436 {
          tunnel: w437 -> [_ w446]
          tunnel: w435 -> [w439 w443]
          tunnel: [w439 w449] -> w434
          frame True {
          }
          frame False {
            n187 = Unbundle By Name(w443) -> ("Sample.GyroZ"=w442:u32)
            n188 = To Unsigned Long Integer(number=w446) -> (unsigned 32bit integer=w445:u32)
            n189 = xnode ("FIFO Method Node")("Element"=w446, "Timeout"=0) -> ()  [unwired: 1 in, 2 out]
            n190 = Logical Shift(y=i16 8, x=w445) -> (x << y=w441:u32)
            n191 = Or(x=w442, y=w441) -> (x .or. y?=w440:u32)
            n192 = Bundle By Name(cluster=w443, "State"=GyroRxLoopStates."ReadSampleZ0" ("t"), "Sample.GyroZ"=w440) -> (w449:T1)
          }
        }
      }
      frame "ReadSampleZ0" {
        n193 = xnode ("FIFO Method Node")("Timeout"=0) -> ("Element"=w453:u8, "Timed Out?"=w452:bool)  [unwired: 1 in, 1 out]
        n194 = case shown="False" w452 {
          tunnel: w453 -> [_ w461]
          tunnel: w451 -> [w455 w460]
          tunnel: [w455 w464] -> w450
          frame True {
          }
          frame False {
            n195 = Unbundle By Name(w460) -> ("Sample.GyroZ"=w459:u32)
            n196 = To Unsigned Long Integer(number=w461) -> (unsigned 32bit integer=w458:u32)
            n197 = xnode ("FIFO Method Node")("Element"=w461, "Timeout"=0) -> ()  [unwired: 1 in, 2 out]
            n198 = Or(x=w459, y=w458) -> (x .or. y?=w457:u32)
            n199 = Bundle By Name(cluster=w460, "State"=GyroRxLoopStates."ReadSampleReserved" ("t"), "Sample.GyroZ"=w457, "ReservedCount"=u8 0) -> (w464:T1)
          }
        }
      }
      frame "ReadSampleReserved" {
        n200 = xnode ("FIFO Method Node")("Timeout"=0) -> ("Element"=w469:u8, "Timed Out?"=w468:bool)  [unwired: 1 in, 1 out]
        n201 = case shown="False" w468 {
          tunnel: w469 -> [_ w480]
          tunnel: w467 -> [w471 w479]
          tunnel: [w471 w482] -> w466
          tunnel: w465 -> [_ w478]
          frame True {
          }
          frame False {
            n202 = Increment(x=w478) -> (x+1=w477:u8)
            n203 = xnode ("FIFO Method Node")("Element"=w480, "Timeout"=0) -> ()  [unwired: 1 in, 2 out]
            n204 = Less?(x=w477, y=u8 12) -> (x < y?=w473:bool)
            n205 = Select(t=GyroRxLoopStates."ReadSampleReserved", s=w473, f=GyroRxLoopStates."ReadSampleStatus") -> (s? t:f=w474:T2)
            n206 = Bundle By Name(cluster=w479, "State"=w474, "ReservedCount"=w477) -> (w482:T1)
          }
        }
      }
      frame "ReadSampleStatus" {
        n207 = xnode ("FIFO Method Node")("Timeout"=0) -> ("Element"=w486:u8, "Timed Out?"=w485:bool)  [unwired: 1 in, 1 out]
        n208 = case shown="False" w485 {
          tunnel: w486 -> [_ w489]
          tunnel: w484 -> [w488 w491]
          tunnel: [w488 w493] -> w483
          frame True {
          }
          frame False {
            n209 = xnode ("FIFO Method Node")("Element"=w489, "Timeout"=0) -> ()  [unwired: 1 in, 2 out]
            n210 = Bundle By Name(cluster=w491, "State"=GyroRxLoopStates."ReadSampleSequenceNumber" ("t"), "Sample.Status"=w489) -> (w493:T1)
          }
        }
      }
      frame "ReadSampleSequenceNumber" {
        n211 = xnode ("FIFO Method Node")("Timeout"=0) -> ("Element"=w497:u8, "Timed Out?"=w496:bool)  [unwired: 1 in, 1 out]
        n212 = case shown="False" w496 {
          tunnel: w497 -> [_ w500]
          tunnel: w495 -> [w499 w502]
          tunnel: [w499 w504] -> w494
          frame True {
          }
          frame False {
            n213 = xnode ("FIFO Method Node")("Element"=w500, "Timeout"=0) -> ()  [unwired: 1 in, 2 out]
            n214 = Bundle By Name(cluster=w502, "State"=GyroRxLoopStates."ReadSampleTemperature1" ("t"), "Sample.SequenceNumber"=w500) -> (w504:T1)
          }
        }
      }
      frame "ReadSampleTemperature1" {
        n215 = xnode ("FIFO Method Node")("Timeout"=0) -> ("Element"=w508:u8, "Timed Out?"=w507:bool)  [unwired: 1 in, 1 out]
        n216 = case shown="False" w507 {
          tunnel: w508 -> [_ w515]
          tunnel: w506 -> [w510 w512]
          tunnel: [w510 w518] -> w505
          frame True {
          }
          frame False {
            n217 = To Word Integer(number=w515) -> (16bit integer=w514:i16)
            n218 = xnode ("FIFO Method Node")("Element"=w515, "Timeout"=0) -> ()  [unwired: 1 in, 2 out]
            n219 = Logical Shift(y=i16 8, x=w514) -> (x << y=w511:i16)
            n220 = Bundle By Name(cluster=w512, "State"=GyroRxLoopStates."ReadSampleTemperature0" ("t"), "Sample.Temperature"=w511) -> (w518:T1)
          }
        }
      }
      frame "ReadSampleTemperature0" {
        n221 = xnode ("FIFO Method Node")("Timeout"=0) -> ("Element"=w522:u8, "Timed Out?"=w521:bool)  [unwired: 1 in, 1 out]
        n222 = case shown="False" w521 {
          tunnel: w522 -> [_ w529]
          tunnel: w520 -> [w524 w528]
          tunnel: [w524 w532] -> w519
          frame True {
          }
          frame False {
            n223 = Unbundle By Name(w528) -> ("Sample.Temperature"=w527:i16)
            n224 = To Word Integer(number=w529) -> (16bit integer=w526:i16)
            n225 = xnode ("FIFO Method Node")("Element"=w529, "Timeout"=0) -> ()  [unwired: 1 in, 2 out]
            n226 = Or(x=w527, y=w526) -> (x .or. y?=w525:i16)
            n227 = Bundle By Name(cluster=w528, "State"=GyroRxLoopStates."ReadSampleCRC3" ("t"), "Sample.Temperature"=w525) -> (w532:T1)
          }
        }
      }
      frame "ReadSampleCRC3" {
        n228 = xnode ("FIFO Method Node")("Timeout"=0) -> ("Element"=w536:u8, "Timed Out?"=w535:bool)  [unwired: 1 in, 1 out]
        n229 = case shown="False" w535 {
          tunnel: w536 -> [_ w545]
          tunnel: w534 -> [w538 w542]
          tunnel: [w538 w547] -> w533
          frame True {
          }
          frame False {
            n230 = To Unsigned Long Integer(number=w545) -> (unsigned 32bit integer=w544:u32)
            n231 = xnode ("FIFO Method Node")("Element"=TRUE, "Timeout"=0) -> ()  [unwired: 1 in, 2 out]
            n232 = Logical Shift(y=i16 24, x=w544) -> (x << y=w541:u32)
            n233 = Bundle By Name(cluster=w542, "State"=GyroRxLoopStates."ReadSampleCRC2" ("t"), "CRC"=w541) -> (w547:T1)
          }
        }
      }
      frame "ReadSampleCRC2" {
        n234 = xnode ("FIFO Method Node")("Timeout"=0) -> ("Element"=w552:u8, "Timed Out?"=w551:bool)  [unwired: 1 in, 1 out]
        n235 = case shown="False" w551 {
          tunnel: w552 -> [_ w561]
          tunnel: w550 -> [w554 w560]
          tunnel: [w554 w563] -> w549
          tunnel: w548 -> [_ w558]
          frame True {
          }
          frame False {
            n236 = To Unsigned Long Integer(number=w561) -> (unsigned 32bit integer=w557:u32)
            n237 = Logical Shift(y=i16 16, x=w557) -> (x << y=w555:u32)
            n238 = Or(x=w558, y=w555) -> (x .or. y?=w559:u32)
            n239 = Bundle By Name(cluster=w560, "State"=GyroRxLoopStates."ReadSampleCRC1" ("t"), "CRC"=w559) -> (w563:T1)
          }
        }
      }
      frame "ReadSampleCRC1" {
        n240 = xnode ("FIFO Method Node")("Timeout"=0) -> ("Element"=w568:u8, "Timed Out?"=w567:bool)  [unwired: 1 in, 1 out]
        n241 = case shown="False" w567 {
          tunnel: w568 -> [_ w577]
          tunnel: w566 -> [w570 w576]
          tunnel: [w570 w579] -> w565
          tunnel: w564 -> [_ w574]
          frame True {
          }
          frame False {
            n242 = To Unsigned Long Integer(number=w577) -> (unsigned 32bit integer=w573:u32)
            n243 = Logical Shift(y=i16 8, x=w573) -> (x << y=w571:u32)
            n244 = Or(x=w574, y=w571) -> (x .or. y?=w575:u32)
            n245 = Bundle By Name(cluster=w576, "State"=GyroRxLoopStates."ReadSampleCRC0" ("t"), "CRC"=w575) -> (w579:T1)
          }
        }
      }
      frame "ReadSampleCRC0" {
        n246 = xnode ("FIFO Method Node")("Timeout"=0) -> ("Element"=w584:u8, "Timed Out?"=w583:bool)  [unwired: 1 in, 1 out]
        n247 = case shown="False" w583 {
          tunnel: w584 -> [_ w591]
          tunnel: w582 -> [w586 w590]
          tunnel: [w586 w593] -> w581
          tunnel: w580 -> [_ w588]
          frame True {
          }
          frame False {
            n248 = To Unsigned Long Integer(number=w591) -> (unsigned 32bit integer=w587:u32)
            n249 = Or(x=w588, y=w587) -> (x .or. y?=w589:u32)
            n250 = Bundle By Name(cluster=w590, "State"=GyroRxLoopStates."VerifyCRC" ("t"), "CRC"=w589) -> (w593:T1)
          }
        }
      }
      frame "VerifyCRC" {
        n251 = xnode ("FIFO Method Node")("Timeout"=0) -> ("Element"=w598:u32, "Timed Out?"=w597:bool)  [unwired: 1 in, 1 out]
        n252 = case shown="False" w597 {
          tunnel: w598 -> [_ w605]
          tunnel: w596 -> [w600 w607]
          tunnel: [w600 w608] -> w595
          tunnel: w594 -> [_ w606]
          frame True {
          }
          frame False {
            n253 = Equal?(x=w606, y=w605) -> (x = y?=w601:bool)
            n254 = case shown="True" w601 {
              frame False {
              }
              frame True {
                n255 = xnode ("Register Read")() -> ("Data"=w610:u64)  [unwired: 1 in, 1 out]
                n256 = Increment(x=w610) -> (x+1=w609:u64)
                n257 = xnode ("Register Write")("Data"=w609) -> ()  [unwired: 1 in, 1 out]
              }
            }
            n258 = Select(t=GyroRxLoopStates."PrepareSample", s=w601, f=GyroRxLoopStates."ResponseCRCError" ("t")) -> (s? t:f=w602:T2)
            n259 = Bundle By Name(cluster=w607, "State"=w602) -> (w608:T1)
          }
        }
      }
      frame "PrepareSample" {
        n260 = xnode ("Register Read")() -> ("Data"=w614:u64)  [unwired: 1 in, 1 out]
        n261 = xnode ("Register Read")() -> ("Data"=w613:u64)  [unwired: 1 in, 1 out]
        n262 = xnode ("Register Read")() -> ("Data"=w612:u64)  [unwired: 1 in, 1 out]
        n263 = xnode ("Register Read")() -> ("Data"=w611:u64)  [unwired: 1 in, 1 out]
        n264 = Bundle By Name(cluster=w618, "State"=GyroRxLoopStates."MoveSample", "Sample.Timestamp"=w615, "Sample.TxBytes"=w614, "Sample.RxBytes"=w613, "Sample.TxFrames"=w612, "Sample.RxFrames"=w611) -> (w617:T1)
      }
      frame "MoveSample" {
        n265 = xnode ("FIFO Method Node")("Element"=w620, "Timeout"=0) -> ()  [unwired: 1 in, 2 out]
        n266 = Bundle By Name(cluster=w623, "State"=GyroRxLoopStates."ClearCRC") -> (w622:T1)
      }
      frame "ResponseHeaderError" {
        n267 = Bundle By Name(cluster=w627, "State"=GyroRxLoopStates."PrepareErrorCode", "ErrorSample.ErrorCode"=GyroErrorCodes."ResponseHeaderError" ("GyroErrorCodes")) -> (w626:T1)
      }
      frame "ResponseCRCError" {
        n268 = Bundle By Name(cluster=w631, "State"=GyroRxLoopStates."PrepareErrorCode", "ErrorSample.ErrorCode"=GyroErrorCodes."ResponseCRCError" ("GyroErrorCodes")) -> (w630:T1)
      }
      frame "ResponseTimeoutError" {
        n269 = Bundle By Name(cluster=w635, "State"=GyroRxLoopStates."PrepareErrorCode", "ErrorSample.ErrorCode"=GyroErrorCodes."ResponseTimeoutError" ("GyroErrorCodes")) -> (w634:T1)
      }
      frame "ResponseChecksumError" {
        n270 = Bundle By Name(cluster=w639, "State"=GyroRxLoopStates."PrepareErrorCode", "ErrorSample.ErrorCode"=GyroErrorCodes."ResponseChecksumError" ("GyroErrorCodes")) -> (w638:T1)
      }
      frame "PrepareErrorCode" {
        n271 = xnode ("Register Read")() -> ("Data"=w643:u64)  [unwired: 1 in, 1 out]
        n272 = xnode ("Register Read")() -> ("Data"=w642:u64)  [unwired: 1 in, 1 out]
        n273 = xnode ("Register Read")() -> ("Data"=w641:u64)  [unwired: 1 in, 1 out]
        n274 = xnode ("Register Read")() -> ("Data"=w640:u64)  [unwired: 1 in, 1 out]
        n275 = Bundle By Name(cluster=w647, "State"=GyroRxLoopStates."MoveErrorCode", "ErrorSample.Timestamp"=w644, "ErrorSample.TxBytes"=w643, "ErrorSample.RxBytes"=w642, "ErrorSample.TxFrames"=w641, "ErrorSample.RxFrames"=w640) -> (w646:T1)
      }
      frame "MoveErrorCode" {
        n276 = xnode ("FIFO Method Node")("Element"=w649, "Timeout"=0) -> ()  [unwired: 1 in, 2 out]
        n277 = Bundle By Name(cluster=w652, "State"=GyroRxLoopStates."ClearCRC") -> (w651:T1)
      }
      frame "ClearCRC" {
        n278 = xnode ("FIFO Method Node")("Element"=TRUE, "Timeout"=0) -> ()  [unwired: 1 in, 2 out]
        n279 = Bundle By Name(cluster=w657, "State"=GyroRxLoopStates."WaitForCRCCleared") -> (w656:T1)
      }
      frame "WaitForCRCCleared" {
        n280 = xnode ("FIFO Method Node")("Timeout"=0) -> ("Timed Out?"=w661:bool)  [unwired: 1 in, 2 out]
        n281 = Select(t=GyroRxLoopStates."WaitForCRCCleared", s=w661, f=GyroRxLoopStates."ReadHeader3" ("State")) -> (s? t:f=w658:T2)
        n282 = Bundle By Name(cluster=w664, "State"=w658) -> (w663:T1)
      }
    }
  }
  n283 = node-c288(w2) -> ()
